vi "array_mem_operation1.vi"() -> ()   [LabVIEW 2019]
uses:
  <vilib>/Analysis/1siggen.llb/General Aperiodic Triangle.vi
  <vilib>/Analysis/NI_AALBase.lvlib
panel:
  in  "stop":bool
  out "Waveform Graph":dbl[](graph)
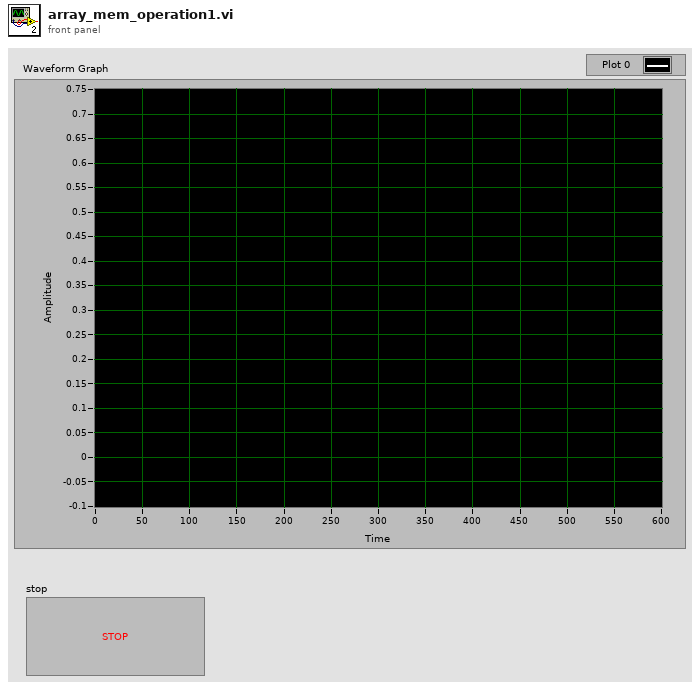
[diagram p1: front panel]
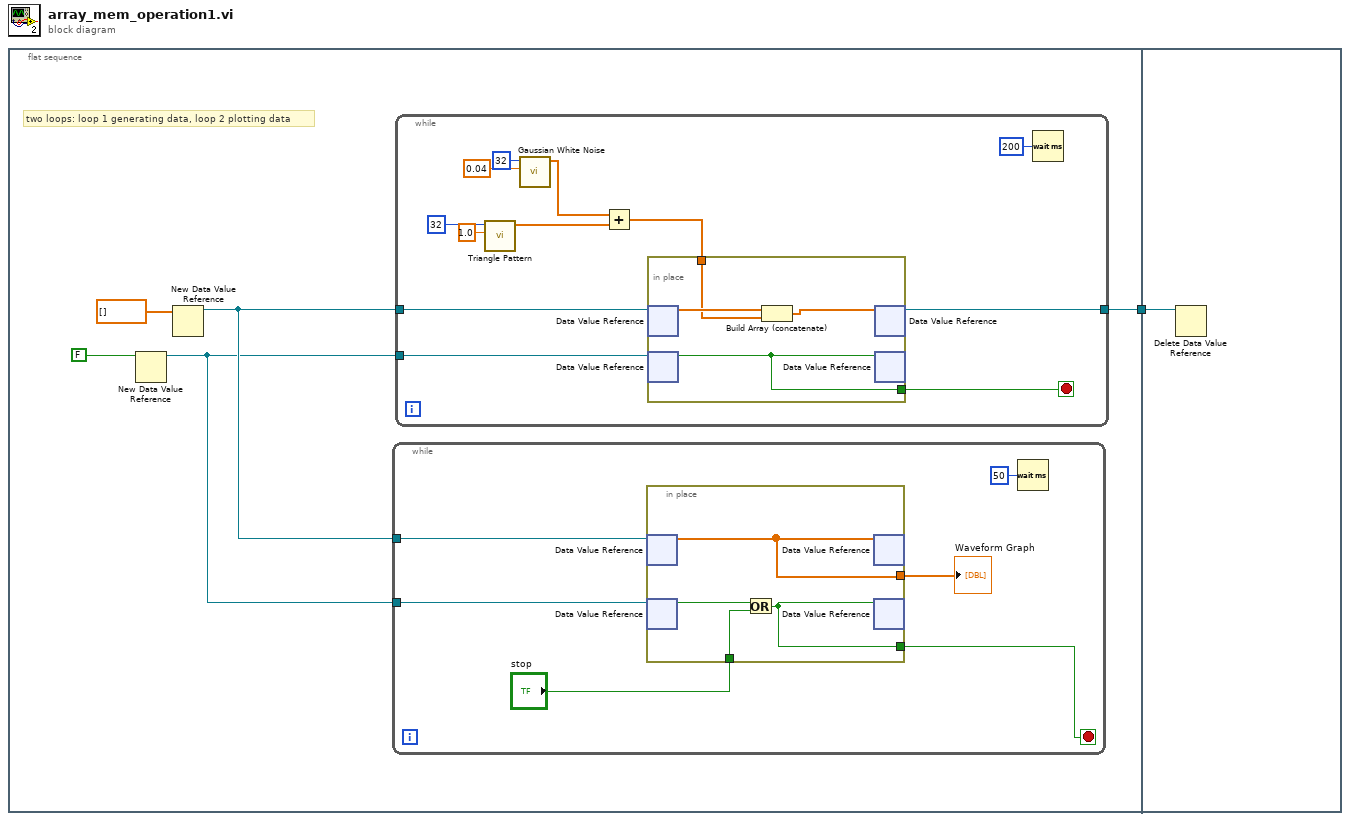
[diagram p0: block diagram]
diagram:
  n1 = flat-sequence {
    tunnel: [w4] -> w1
    tunnel: w1 -> [w33]
    frame #0 {
      # "two loops: loop 1 generating data, loop 2 plotting data"
      n2 = New Data Value Reference(data value=FALSE) -> (data value reference=w2:refnum<data-value>)  [unwired: 1 in, 1 out]
      n3 = New Data Value Reference(data value=dbl[] []) -> (data value reference=w5:refnum<data-value>)  [unwired: 1 in, 1 out]
      n4 = while {
        tunnel: w5 -> [w12]
        tunnel: w2 -> [w9]
        stop <- w7 stop-if-true
        n5 = in-place {
          in-place-border: [w16] -> w11
          in-place-border: "stop" -> [w14]
          in-place-border: [w13] -> w7
          n6 = in-place-dvr #1(w12) -> (w16:dbl[])  [unwired: 1 out]
          n7 = in-place-dvr #2(w9) -> (w15:bool)  [unwired: 1 out]
          n8 = Or(x=w15, y=w14) -> (x .or. y?=w13:bool)
          n9 = in-place-dvr #1(w16) -> ()  [unwired: 2 out]
          n10 = in-place-dvr #2(w13) -> ()  [unwired: 2 out]
        }
        "Waveform Graph" <- w11
        n11 = Wait (ms)(milliseconds to wait=u32 50) -> ()  [unwired: 1 out]
      }
      n12 = while {
        tunnel: w5 -> [w22]
        tunnel: [w19] -> w4
        tunnel: w2 -> [w18]
        stop <- w17 stop-if-true
        n13 = call <vilib>:"Triangle Pattern.vi"("amplitude"=1.0, "samples"=32) -> ("Triangle Pattern"=w23:dbl[])  [unwired: 8 in, 1 out]
        n14 = call <vilib>:"Gaussian White Noise.vi"("standard deviation"=0.04, "samples"=32) -> ("Gaussian noise pattern"=w24:dbl[])  [unwired: 8 in, 1 out]
        n15 = Add(x=w24, y=w23) -> (x+y=w20:dbl[])
        n16 = in-place {
          in-place-border: w20 -> [w31]
          in-place-border: [w29] -> w17
          n17 = in-place-dvr #3(w22) -> (w32:dbl[])  [unwired: 1 out]
          n18 = in-place-dvr #4(w18) -> (w29:bool)  [unwired: 1 out]
          n19 = Build Array (concatenate)(w32, w31) -> (w30:dbl[])
          n20 = in-place-dvr #3(w30) -> (w19:refnum<data-value>)  [unwired: 1 out]
          n21 = in-place-dvr #4(w29) -> ()  [unwired: 2 out]
        }
        n22 = Wait (ms)(milliseconds to wait=u32 200) -> ()  [unwired: 1 out]
      }
    }
    frame #1 {
      n23 = Delete Data Value Reference(data value reference=w33) -> ()  [unwired: 1 in, 2 out]
    }
  }
